vi "GetProperties.vi"(8 "error in":errorcluster, 11 "ColorScale in":refnum<class "ColorScale.lvclass">) -> (0 "error out":errorcluster, 3 "ColorScale out":refnum<class "ColorScale.lvclass">)   [LabVIEW 2014, in "Raspberry Pi Compatible Compiler for LabVIEW.lvlib" / "ColorScale.lvclass"]
uses:
  ColorScale.lvclass
  ColorScale.lvclass/ColorScale.ctl
  Scale/Scale.lvclass
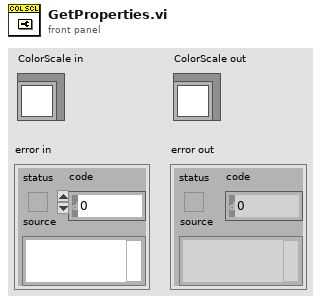
[diagram p1: front panel]
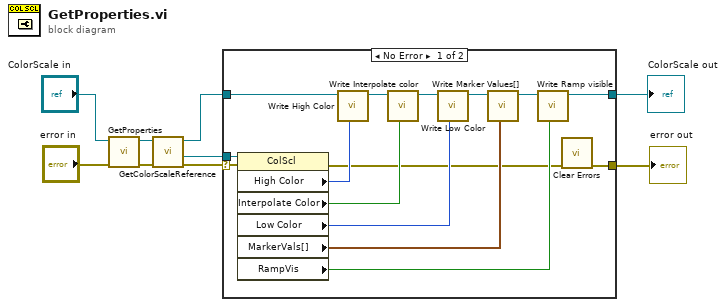
[diagram p0: block diagram]
diagram:
  n1 = call-parent "GetProperties.vi"("error in"="error in", "Scale in"="ColorScale in") -> ("error out"=w6:errorcluster, "Scale out"=w7:refnum<class "ColorScale.lvclass">)  [unwired: 8 in]
  n2 = call "GetColorScaleReference.vi"("error in"=w6, "ColorScale in"=w7) -> ("error out"=w5:errorcluster, "color scale reference"=w4:refnum<vi>, "ColorScale out"=w3:refnum<class "ColorScale.lvclass">)  [unwired: 7 in]
  n3 = case shown="No Error" w5 {
    selector: w5 -> [w23 w25]
    tunnel: w4 -> [w24 _]
    tunnel: w3 -> [w17 w26]
    tunnel: [w10 w25] -> w1
    tunnel: [w15 w26] -> w2
    frame No Error {
      n4 = property class="ColScl"(reference=w24, error in=w23) -> (error out=w16:errorcluster, "High Color"=w22:u32, "Interpolate Color"=w21:bool, "Low Color"=w20:u32, "MarkerVals[]"=w19:cluster{dbl, u32}[], "RampVis"=w18:bool)  [unwired: 1 out]
      n5 = call "Write High Color.vi"("High Color"=w22, "ColorScale in"=w17) -> ("ColorScale out"=w11:refnum<class "ColorScale.lvclass">)  [unwired: 7 in]
      n6 = call "Write Interpolate color.vi"("Interpolate color"=w21, "ColorScale in"=w11) -> ("ColorScale out"=w12:refnum<class "ColorScale.lvclass">)  [unwired: 7 in]
      n7 = call "Write Low Color.vi"("Low Color"=w20, "ColorScale in"=w12) -> ("ColorScale out"=w13:refnum<class "ColorScale.lvclass">)  [unwired: 7 in]
      n8 = call "Write Marker Values[].vi"("Marker Values[]"=w19, "ColorScale in"=w13) -> ("ColorScale out"=w14:refnum<class "ColorScale.lvclass">)  [unwired: 7 in]
      n9 = call "Write Ramp visible.vi"("Ramp visible"=w18, "ColorScale in"=w14) -> ("ColorScale out"=w15:refnum<class "ColorScale.lvclass">)  [unwired: 7 in]
      n10 = call <vilib>:"Clear Errors.vi"("error in (no error)"=w16) -> ("error out"=w10:errorcluster)  [unwired: 5 in, 1 out]
    }
    frame Error {
    }
  }
  "error out" <- w1
  "ColorScale out" <- w2
